vi "6133_N采样.vi"(2 "率":dbl=64000.0, 3 "采样数":i32=64000, 4 "timeout (s)":dbl=10.0 caption="超时(s)" format="%0.2f", 5 "error in":errorcluster caption="错误输入", 10 "设备名":tag="6133") -> (15 "data":dbl[][](array[numeric]) caption="数据" format="%0.2f", 19 "error out":errorcluster caption="错误输出")   [LabVIEW 2014]
doc: "通过NI-DAQmx创建、编辑和运行任务。关于NI-DAQmx支持设备的完整列表，见NI-DAQ自述文件。\n\n在程序框图上放置DAQ助手Express VI，可通过DAQ助手新建任务。创建任务后，双击DAQ助手Express VI可编辑该任务。如需连续进行测量或信号生成，可将DAQ助手Express VI置于While循环内。"
uses:
  <vilib>/DAQmx/read.llb/DAQmx Read.vi
  <vilib>/DAQmx/read.llb/DAQmx Read (Analog 2D DBL NChan NSamp).vi
  <vilib>/DAQmx/miscellaneous.llb/DAQmx Fill In Error Info.vi
  <vilib>/DAQmx/configure/timing.llb/DAQmx Timing (Sample Clock).vi
  <vilib>/DAQmx/create/channels.llb/DAQmx Create Channel (AI-Voltage-Basic).vi
  <vilib>/DAQmx/create/channels.llb/DAQmx Create Channel (TEDS-AI-Voltage-Basic).vi
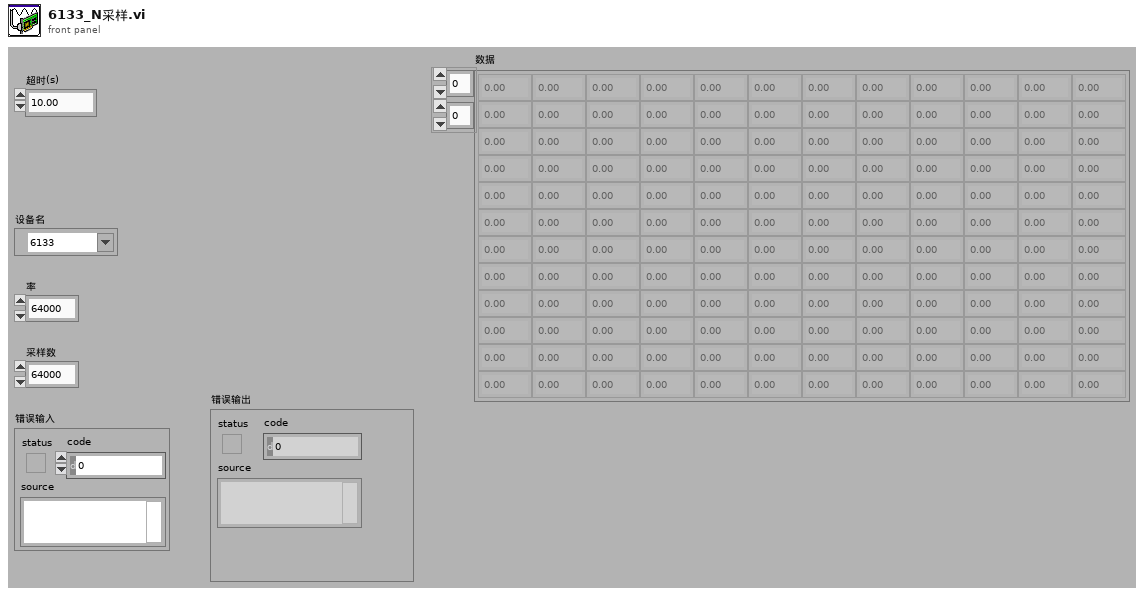
[diagram p1: front panel]
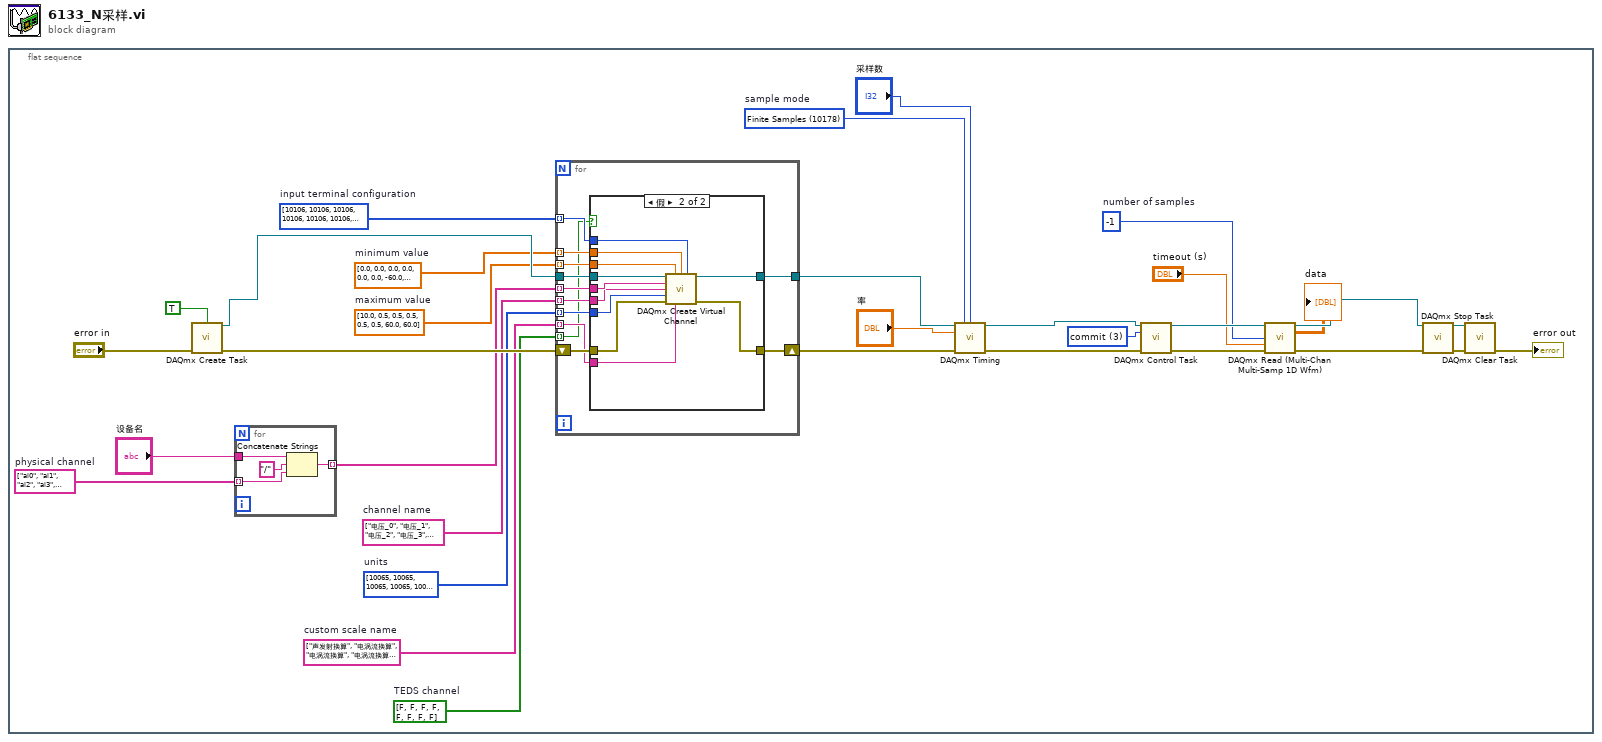
[diagram p0: block diagram]
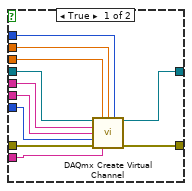
[diagram p2: hidden frame]
diagram:
  n1 = flat-sequence {
    frame #0 {
      w1 = i32[] [10106, 10106, 10106, 10106, 10106, 10106, 10106, 10106] items=["default"=-1, "RSE"=10083, "NRSE"=10078, "Differential"=10106, "Pseudodifferential"=12529]  # input terminal configuration
      w2 = dbl[] [10.0, 0.5, 0.5, 0.5, 0.5, 0.5, 60.0, 60.0]  # maximum value
      w3 = dbl[] [0.0, 0.0, 0.0, 0.0, 0.0, 0.0, -60.0, -60.0]  # minimum value
      w4 = string[] ["电压_0", "电压_1", "电压_2", "电压_3", "电压_4", "电压_5", "电压_6", "电压_7"]  # channel name
      w5 = i32[] [10065, 10065, 10065, 10065, 10065, 10065, 10065, 10065] items=["Volts"=10348, "From TEDS"=12516, "From Custom Scale"=10065]  # units
      w6 = string[] ["声发射换算", "电涡流换算", "电涡流换算", "电涡流换算", "电涡流换算", "电涡流换算", "加速度换算", "加速度换算"]  # custom scale name
      w9 = 3 items=["verify"=2, "reserve"=4, "commit"=3, "unreserve"=5, "abort"=6] ("action")
      w15 = -1  # number of samples
      w20 = 10178 items=["Finite Samples"=10178, "Continuous Samples"=10123, "Hardware Timed Single Point"=12522]  # sample mode
      w25 = bool[] [FALSE, FALSE, FALSE, FALSE, FALSE, FALSE, FALSE, FALSE]  # TEDS channel
      w29 = string[] ["ai0", "ai1", "ai2", "ai3", "ai4", "ai5", "ai6", "ai7"]  # physical channel
      n2 = call <vilib>:"DAQmx Create Task.vi"("auto cleanup"=TRUE, "error in"="error in") -> ("task out"=w28:refnum<k21>, "error out"=w27:errorcluster)  [unwired: 12 in]
      n3 = for "For循环" {
        tunnel: [w36] -> w26 mode=indexing
        tunnel: "设备名" -> [w35]
        tunnel: w29 -> [w33] mode=indexing
        n4 = Concatenate Strings(w35, "/" ("string"), w33) -> (w36:string)
      }
      n5 = for "For循环" {
        tunnel: w28 -> [w48]
        tunnel: [w46] -> w24
        tunnel: w1 -> [w44] mode=indexing
        tunnel: w3 -> [w43] mode=indexing
        tunnel: w2 -> [w42] mode=indexing
        tunnel: w26 -> [w41] mode=indexing
        tunnel: w4 -> [w40] mode=indexing
        tunnel: w5 -> [w39] mode=indexing
        tunnel: w6 -> [w38] mode=indexing
        shift-right: [w45] -> w23
        shift-left: w27 -> [w47]
        tunnel: w25 -> [w37] mode=indexing
        n6 = case "条件结构" shown="假" w37 {
          tunnel: w48 -> [w59 w70]
          tunnel: w47 -> [w58 w69]
          tunnel: [w57 w68] -> w46
          tunnel: [w56 w60] -> w45
          tunnel: w44 -> [w55 w67]
          tunnel: w43 -> [w54 w66]
          tunnel: w42 -> [w53 w65]
          tunnel: w41 -> [w52 w64]
          tunnel: w40 -> [w51 w63]
          tunnel: w39 -> [w50 w62]
          tunnel: w38 -> [w49 w61]
          frame True {
            n7 = call-poly <vilib>:"DAQmx Create Virtual Channel.vi"("task in"=w59, "maximum value"=w53, "minimum value"=w54, "input terminal configuration"=w55, "physical channels"=w52, "name to assign"=w51, "units"=w50, "error in"=w58, "custom scale name"=w49) -> ("task out"=w57:refnum<k21>, "error out"=w56:errorcluster)  [unwired: 5 in]
          }
          frame False {
            n8 = call-poly <vilib>:"DAQmx Create Virtual Channel.vi"("task in"=w70, "maximum value"=w65, "minimum value"=w66, "input terminal configuration"=w67, "physical channels"=w64, "name to assign"=w63, "units"=w62, "error in"=w69, "custom scale name"=w61) -> ("task out"=w68:refnum<k21>, "error out"=w60:errorcluster)  [unwired: 5 in]
          }
        }
      }
      n9 = call-poly <vilib>:"DAQmx Timing.vi"("task/channels in"=w24, "sample mode"=w20, "samples per channel"="采样数", "rate"="率", "error in"=w23) -> ("task out"=w19:refnum<k21>, "error out"=w18:errorcluster)  [unwired: 9 in]
      n10 = call <vilib>:"DAQmx Control Task.vi"("task/channels in"=w19, "action"=w9, "error in"=w18) -> ("task out"=w17:refnum<k21>, "error out"=w16:errorcluster)  [unwired: 11 in]
      n11 = call-poly "DAQmx Read (Multi-Chan Multi-Samp 1D Wfm).vi"("task/channels in"=w17, "number of samples per channel"=w15, "timeout"="timeout (s)", "error in"=w16) -> ("task out"=w13:refnum<k21>, "data"=→"data":dbl[][], "error out"=w12:errorcluster)  [unwired: 9 in]
      n12 = call <vilib>:"DAQmx Stop Task.vi"("task/channels in"=w13, "error in"=w12) -> ("task out"=w7:refnum<k21>, "error out"=w8:errorcluster)  [unwired: 12 in]
      n13 = call <vilib>:"DAQmx Clear Task.vi"("task in"=w7, "error in"=w8) -> ("error out"=→"error out":errorcluster)  [unwired: 13 in]
    }
  }
